vi "Initialize.vi"(8 "error in (no error)":errorcluster, 11 "Trigger in":refnum<class "Trigger.lvclass">) -> (0 "error out":errorcluster, 3 "Trigger out":refnum<class "Trigger.lvclass">)   [LabVIEW 2015, in "Waveform Data Logger Engine.lvlib" / "Trigger.lvclass"]
uses:
  Trigger.lvclass
  Trigger.lvclass/Trigger.ctl
  Digital Edge Trigger/Digital Edge Trigger.lvclass
  Digital Edge Trigger/Digital Edge Trigger.lvclass/Digital Edge Trigger.ctl
  Analog Edge Trigger/Analog Edge Trigger.lvclass
  Analog Edge Trigger/Analog Edge Trigger.lvclass/Analog Edge Trigger.ctl
  Value Change Trigger/Value Change Trigger.lvclass
  Value Change Trigger/Value Change Trigger.lvclass/Value Change Trigger.ctl
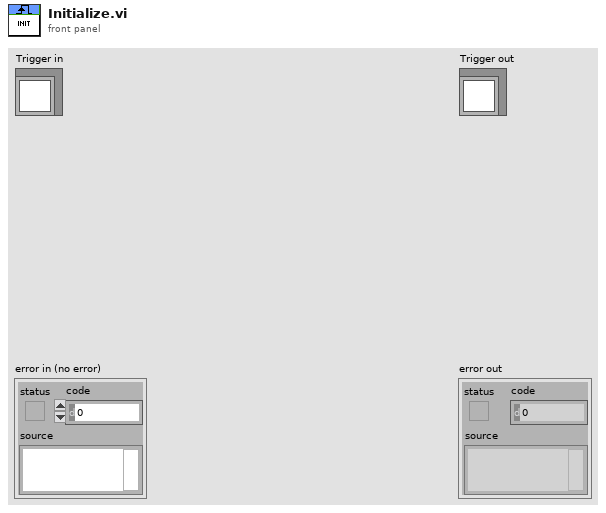
[diagram p1: front panel]
types:
  T1 = typedef "Waveform Data Logger Engine.lvlib/Trigger.lvclass/Trigger Type.ctl" = enum16{"Default", "Digital Edge", "Analog Edge", "In Range", "Value Change", "Boolean Evaluation"}
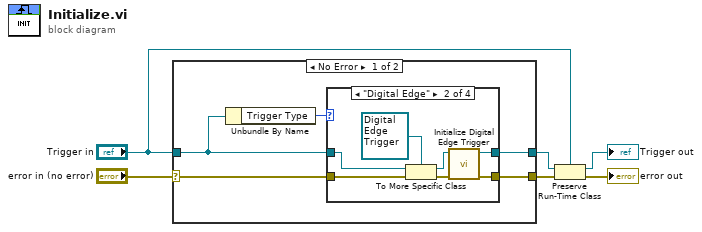
[diagram p0: block diagram]
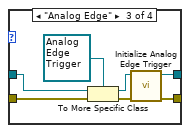
[diagram p3: hidden frame]
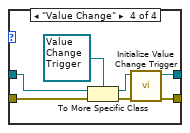
[diagram p4: hidden frame]
diagram:
  n1 = case shown="No Error" "error in (no error)" {
    selector: "error in (no error)" -> [w8 w35]
    tunnel: "Trigger in" -> [w10 w36]
    tunnel: [w9 w36] -> w2
    tunnel: [w7 w35] -> w5
    frame No Error {
      n2 = Unbundle By Name(w10) -> ("Trigger Type"=w11:T1)
      n3 = case shown="\"Digital Edge\"" w11 {
        tunnel: w10 -> [w13 w18 w27 w34]
        tunnel: [w13 w20 w21 w28] -> w9
        tunnel: [w12 w15 w23 w30] -> w7
        tunnel: w8 -> [w12 w14 w26 w33]
        frame Default {
        }
        frame "Digital Edge" {
          n4 = To More Specific Class(target class=refnum<class "Digital Edge Trigger.lvclass"> refnum ("Digital Edge Trigger.lvclass"), reference=w18, error in=w14) -> (specific class reference=w16:refnum<class "Digital Edge Trigger.lvclass">, error out=w19:errorcluster)
          n5 = call "Initialize Digital Edge Trigger.vi"("error in (no error)"=w19, "Digital Edge Trigger in"=w16) -> ("error out"=w15:errorcluster, "Digital Edge Trigger out"=w20:refnum<class "Digital Edge Trigger.lvclass">)  [unwired: 8 in]
        }
        frame "Analog Edge" {
          n6 = To More Specific Class(target class=refnum<class "Analog Edge Trigger.lvclass"> refnum ("Analog Edge Trigger.lvclass"), reference=w27, error in=w26) -> (specific class reference=w22:refnum<class "Analog Edge Trigger.lvclass">, error out=w24:errorcluster)
          n7 = call "Initialize Analog Edge Trigger.vi"("error in (no error)"=w24, "Analog Edge Trigger in"=w22) -> ("error out"=w23:errorcluster, "Analog Edge Trigger out"=w21:refnum<class "Analog Edge Trigger.lvclass">)  [unwired: 8 in]
        }
        frame "Value Change" {
          n8 = To More Specific Class(target class=refnum<class "Value Change Trigger.lvclass"> refnum ("Value Change Trigger.lvclass"), reference=w34, error in=w33) -> (specific class reference=w29:refnum<class "Value Change Trigger.lvclass">, error out=w31:errorcluster)
          n9 = call "Initialize Value Change Trigger.vi"("error in (no error)"=w31, "Value Change Trigger in"=w29) -> ("error out"=w30:errorcluster, "Value Change Trigger out"=w28:refnum<class "Value Change Trigger.lvclass">)  [unwired: 8 in]
        }
      }
    }
    frame Error {
    }
  }
  n10 = Preserve Run-Time Class(object in=w2, error in=w5, 2:"Trigger in") -> (object out=→"Trigger out":refnum<class "Trigger.lvclass">, error out=→"error out":errorcluster)
